vi "Setup Report Paths.vi"(11 "LUnitCLI in":refnum<class "LUnitCLI.lvclass">) -> (3 "LUnitCLI out":refnum<class "LUnitCLI.lvclass">)   [LabVIEW 2020, in "LUnitCLI.lvclass"]
uses:
  LUnitCLI.lvclass
  LUnitCLI.lvclass/LUnitCLI.ctl
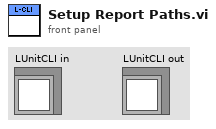
[diagram p1: front panel]
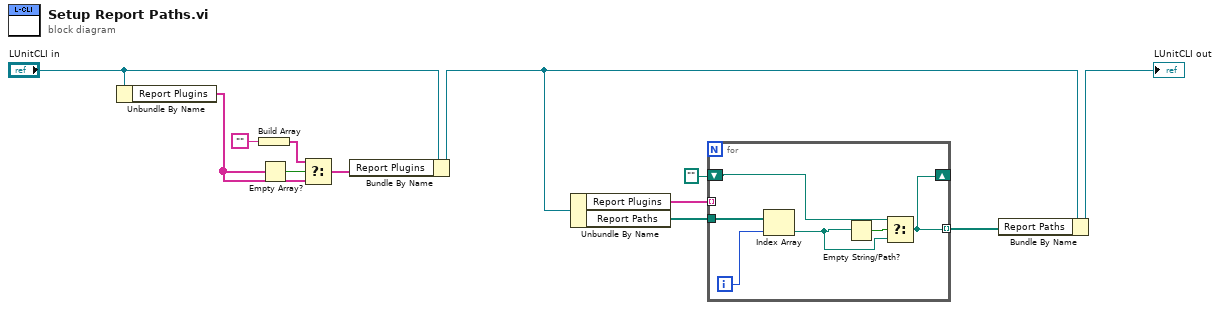
[diagram p0: block diagram]
diagram:
  n1 = Unbundle By Name("LUnitCLI in") -> ("Report Plugins"=w12:string[])
  n2 = Build Array("" ("t")) -> (w10:string[])
  n3 = Empty Array?(array=w12) -> (empty?=w8:bool)
  n4 = Select(t=w10, s=w8, f=w12) -> (s? t:f=w7:string[])
  n5 = Bundle By Name(cluster="LUnitCLI in", "Report Plugins"=w7) -> (w6:refnum<class "LUnitCLI.lvclass">)
  n6 = Unbundle By Name(w6) -> ("Report Plugins"=w5:string[], "Report Paths"=w4:path[])
  n7 = for {
    tunnel: w5 -> [_] mode=indexing
    tunnel: w4 -> [w18]
    shift-right: [w13] -> _
    shift-left: path "" -> [w15]
    tunnel: [w13] -> w1 mode=indexing
    i -> [w17]
    n8 = Index Array(array=w18, index=w17) -> (element=w14:path)
    n9 = Empty String/Path?(string/path=w14) -> (empty?=w16:bool)
    n10 = Select(t=w15, s=w16, f=w14) -> (s? t:f=w13:path)
  }
  n11 = Bundle By Name(cluster=w6, "Report Paths"=w1) -> (→"LUnitCLI out":refnum<class "LUnitCLI.lvclass">)
